vi "SimpleSM.vi"() -> ()   [LabVIEW 2019]
uses:
  States.ctl
  <vilib>/ErrorRing/Error Ring.xnode
panel:
  in  "stop":bool
  out "Waveform Chart":dbl(graph)
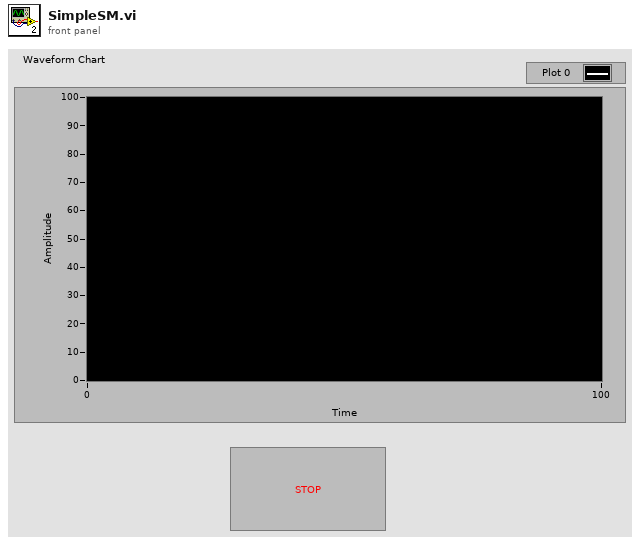
[diagram p1: front panel]
types:
  T1 = typedef "States.ctl" = enum16{"Idle", "DataInitialize", "UIInitialize", "GetData", "CheckRange", "PopUpMessage", "UIUpdate", "Exit"}
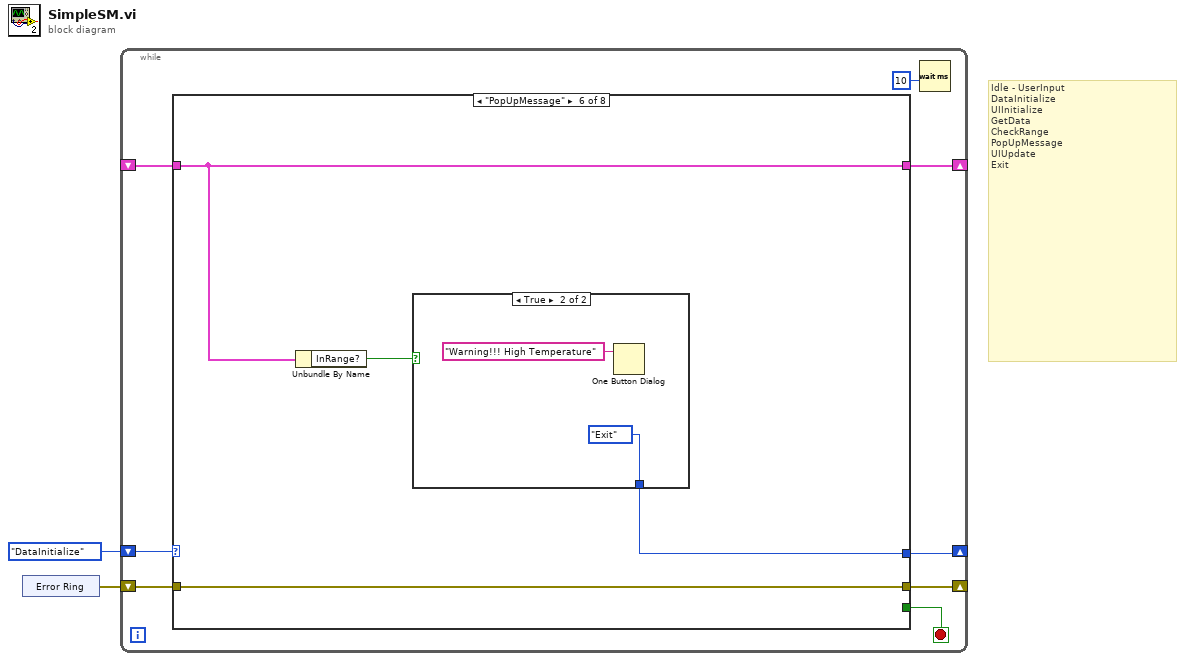
[diagram p0: block diagram]
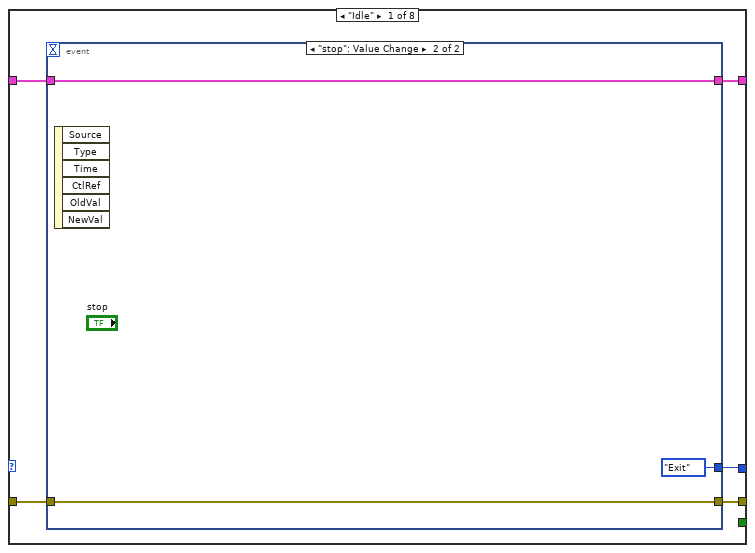
[diagram p2: hidden frame]
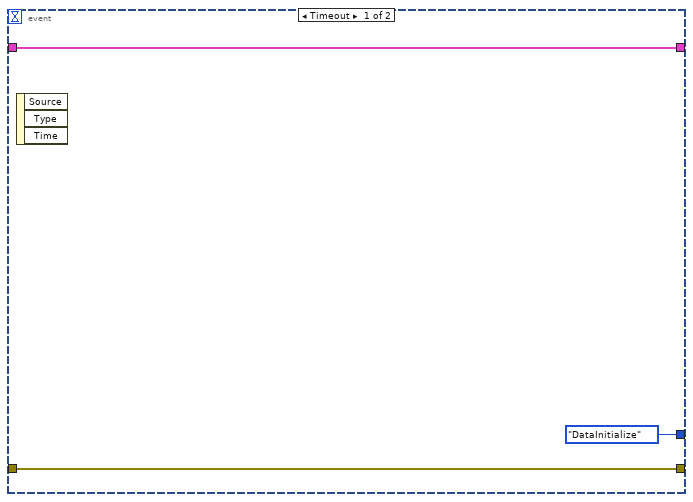
[diagram p3: hidden frame]
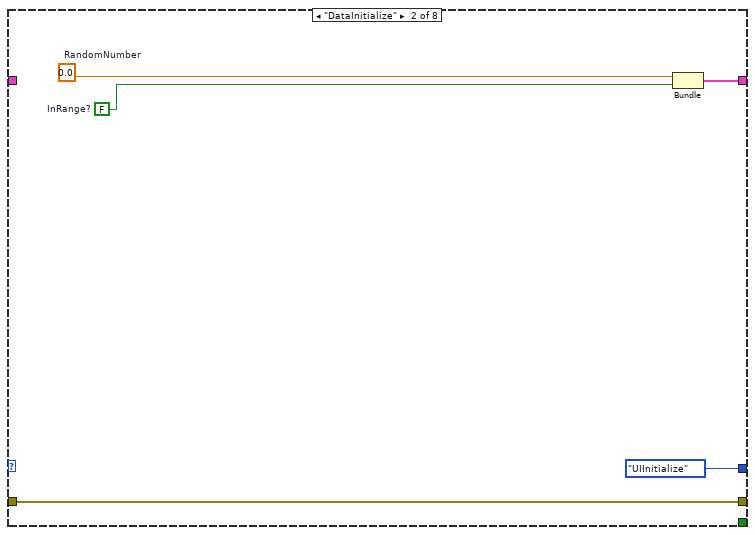
[diagram p4: hidden frame]
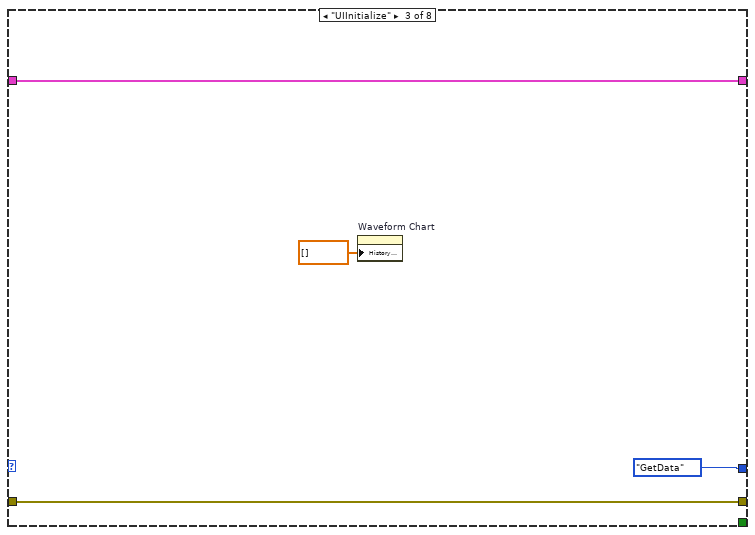
[diagram p5: hidden frame]
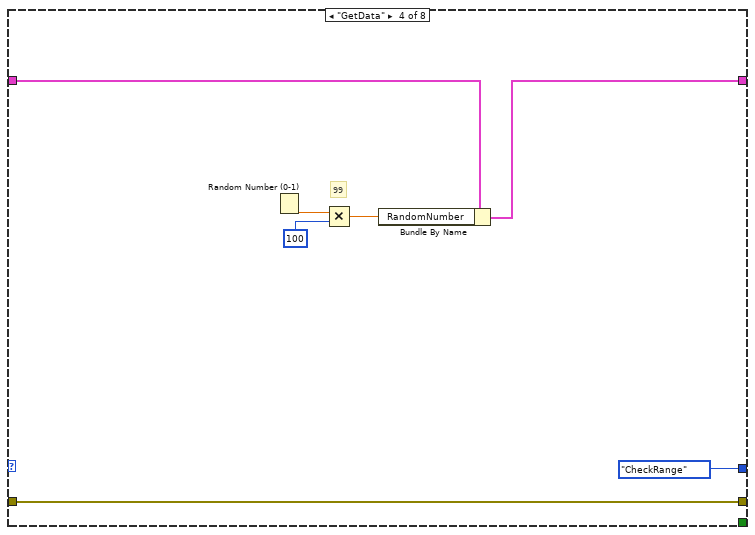
[diagram p6: hidden frame]
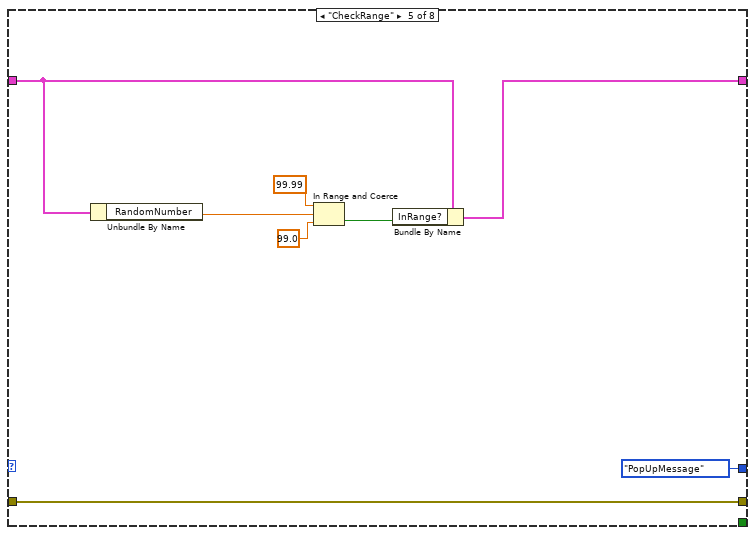
[diagram p7: hidden frame]
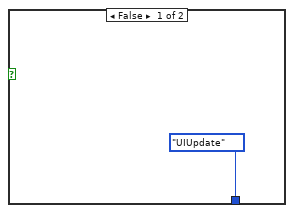
[diagram p8: hidden frame]
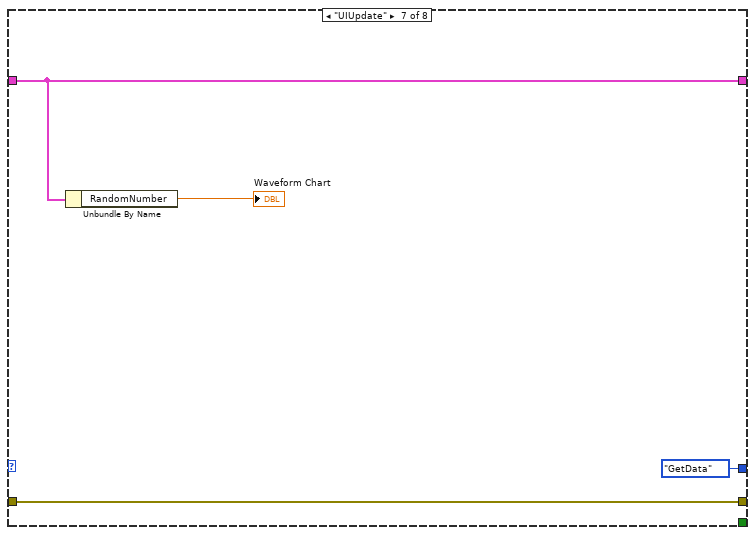
[diagram p9: hidden frame]
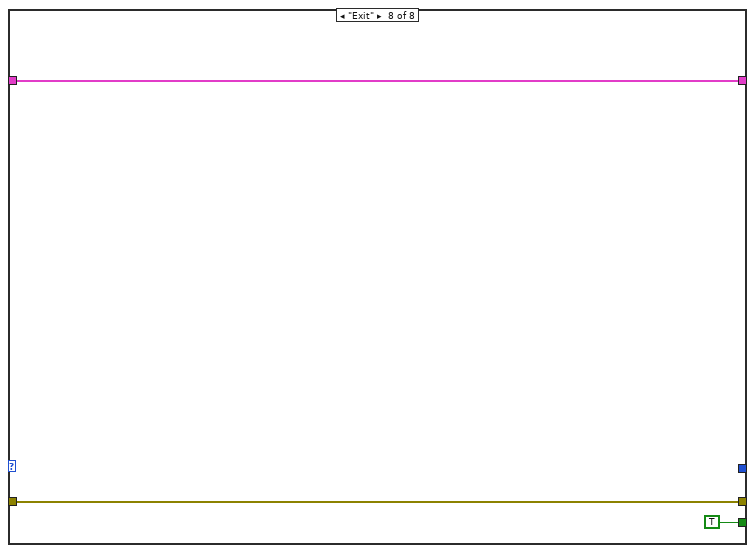
[diagram p10: hidden frame]
diagram:
  # "Idle - UserInput \nDataInitialize\nUIInitialize\nGetData\nCheckRange\nPopUpMessage\nUIUpdate\nExit"
  n1 = xnode "Error Ring"() -> ("error out"=w1:errorcluster)
  n2 = while {
    shift-right: [w5] -> _
    shift-left: States."DataInitialize" -> [w10]
    shift-right: [w7] -> _
    shift-left: w1 -> [w9]
    shift-right: [w8] -> _
    shift-left: _ -> [w6]
    stop <- w4 stop-if-true
    n3 = case shown="\"PopUpMessage\"" w10 {
      tunnel: w9 -> [w15 w24 w30 w37 w45 w49 w56 w59]
      tunnel: [w12 w26 w29 w33 w40 w48 w55 w58] -> w8
      tunnel: [w14 w24 w30 w37 w45 w49 w56 w59] -> w7
      tunnel: w6 -> [w13 _ w29 w32 w39 w48 w55 w58]
      tunnel: [w11 States."UIInitialize" States."GetData" States."CheckRange" States."PopUpMessage" w46 States."GetData" _] -> w5
      tunnel: [_ _ _ _ _ _ _ TRUE] -> w4
      frame "Idle" {
        n4 = event shown="[1] \"stop\": Value Change" {
          selector: _ -> [_ _]
          dyn-events: _ -> [_ _]
          timeout: _ -> [_ _]
          tunnel: w15 -> [w18 w21]
          tunnel: [w18 w21] -> w14
          tunnel: w13 -> [w17 w20]
          tunnel: [w17 w20] -> w12
          tunnel: [States."DataInitialize" States."Exit"] -> w11
          event Timeout {
            n5 = event-data() -> ()  [unwired: 1 in, 3 out]
          }
          event "stop": Value Change {
            n6 = event-data() -> ()  [unwired: 1 in, 6 out]
          }
        }
      }
      frame "DataInitialize" {
        w22 = FALSE  # InRange?
        w25 = 0.0  # RandomNumber
        n7 = Bundle("RandomNumber"=w25, "InRange?"=w22) -> (w26:cluster{"RandomNumber":dbl, "InRange?":bool})  [unwired: 1 in]
      }
      frame "UIInitialize" {
        n8 = property on="Waveform Chart" class="WFChart (strict)"("History Data"=dbl[] []) -> ()  [unwired: 2 in, 2 out]
      }
      frame "GetData" {
        # "99"
        n9 = Random Number (0-1)() -> (number: 0 to 1=w36:dbl)
        n10 = Multiply(x=w36, y=100) -> (x*y=w34:dbl)
        n11 = Bundle By Name(cluster=w32, "RandomNumber"=w34) -> (w33:cluster{"RandomNumber":dbl, "InRange?":bool})
      }
      frame "CheckRange" {
        n12 = Unbundle By Name(w39) -> ("RandomNumber"=w44:dbl)
        n13 = In Range and Coerce(upper limit=99.99, x=w44, lower limit=99.0) -> (In Range?=w41:bool)  [unwired: 1 out]
        n14 = Bundle By Name(cluster=w39, "InRange?"=w41) -> (w40:cluster{"RandomNumber":dbl, "InRange?":bool})
      }
      frame "PopUpMessage" {
        n15 = Unbundle By Name(w48) -> ("InRange?"=w47:bool)
        n16 = case shown="True" w47 {
          tunnel: [States."UIUpdate" States."Exit"] -> w46
          frame False {
          }
          frame True {
            n17 = One Button Dialog(message="Warning!!! High Temperature") -> ()  [unwired: 1 in, 1 out]
          }
        }
      }
      frame "UIUpdate" {
        n18 = Unbundle By Name(w55) -> ("RandomNumber"=→"Waveform Chart":dbl)
      }
      frame "Exit" {
      }
    }
    n19 = Wait (ms)(milliseconds to wait=u32 10) -> ()  [unwired: 1 out]
  }
